vi "logMessages.vi"(11 "State":T1) -> (3 "Output Log":string)   [LabVIEW 2020]
uses:
  controls/State.ctl
  terminal_test.vi
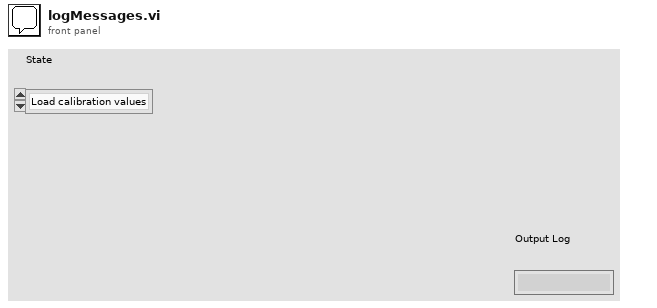
[diagram p1: front panel]
types:
  T1 = typedef "State.ctl" = enum16{"Load calibration values", "Initialize Session", "Initialize TensorFlow Model", "Initialize OBD", "Initialize Image refnum", "Get frame", "Get speed", "Analyze image", "Update reaction space"}
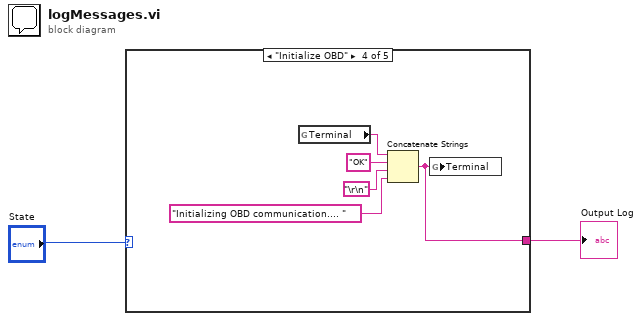
[diagram p0: block diagram]
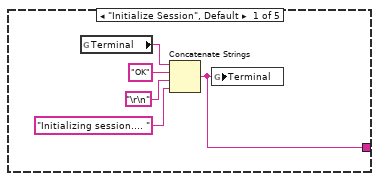
[diagram p2: hidden frame]
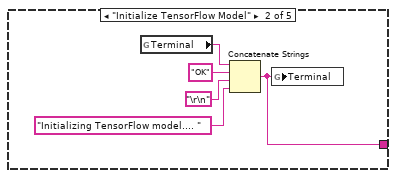
[diagram p3: hidden frame]
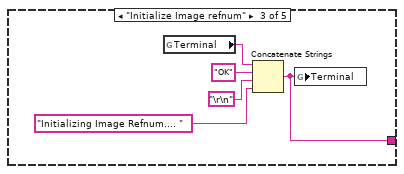
[diagram p4: hidden frame]
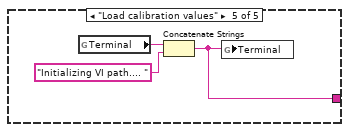
[diagram p5: hidden frame]
diagram:
  n1 = case shown="\"Initialize OBD\"" "State" {
    tunnel: [w3 w8 w13 w18 w23] -> w1
    frame "Initialize Session", Default {
      n2 = global read "terminal_test.vi" "Terminal"() -> (w7:string)
      n3 = Concatenate Strings(w7, "OK", "\r\n", "Initializing session.... ") -> (w3:string)
      n4 = global write "terminal_test.vi" "Terminal"(w3) -> ()
    }
    frame "Initialize TensorFlow Model" {
      n5 = global read "terminal_test.vi" "Terminal"() -> (w12:string)
      n6 = Concatenate Strings(w12, "OK", "\r\n", "Initializing TensorFlow model.... ") -> (w8:string)
      n7 = global write "terminal_test.vi" "Terminal"(w8) -> ()
    }
    frame "Initialize Image refnum" {
      n8 = global read "terminal_test.vi" "Terminal"() -> (w17:string)
      n9 = Concatenate Strings(w17, "OK", "\r\n", "Initializing Image Refnum.... ") -> (w13:string)
      n10 = global write "terminal_test.vi" "Terminal"(w13) -> ()
    }
    frame "Initialize OBD" {
      n11 = global read "terminal_test.vi" "Terminal"() -> (w22:string)
      n12 = Concatenate Strings(w22, "OK", "\r\n", "Initializing OBD communication.... ") -> (w18:string)
      n13 = global write "terminal_test.vi" "Terminal"(w18) -> ()
    }
    frame "Load calibration values" {
      n14 = global read "terminal_test.vi" "Terminal"() -> (w25:string)
      n15 = Concatenate Strings(w25, "Initializing VI path.... ") -> (w23:string)
      n16 = global write "terminal_test.vi" "Terminal"(w23) -> ()
    }
  }
  "Output Log" <- w1
